vi "关键参数查询.vi"() -> ()   [LabVIEW 2016, in "斯坦道总磷.lvlib"]
panel:
  in  "参数下拉列表":u16(ring)
  out "关键参数":T1
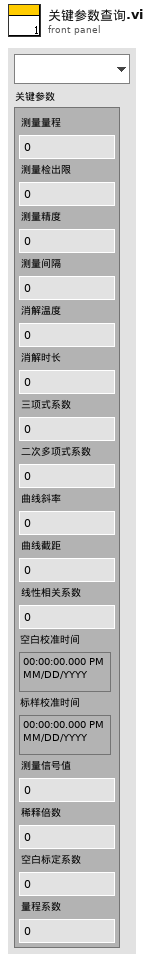
[diagram p1: front panel]
types:
  T1 = typedef "斯坦道总磷.lvlib/关键参数.ctl" = cluster{"测量量程":sgl, "测量检出限":sgl, "测量精度":sgl, "测量间隔":sgl, "消解温度":sgl, "消解时长":sgl, "三项式系数":sgl, "二次多项式系数":sgl, "曲线斜率":sgl, "曲线截距":sgl, "线性相关系数":sgl, "空白校准时间":timestamp, "标样校准时间":timestamp, "测量信号值":sgl, "稀释倍数":sgl, "空白标定系数":sgl, "量程系数":sgl}
  T2 = typedef "LVStringsAndValuesArrayTypeDef_U16.ctl" = cluster{"String":string, "Value":u16}[]
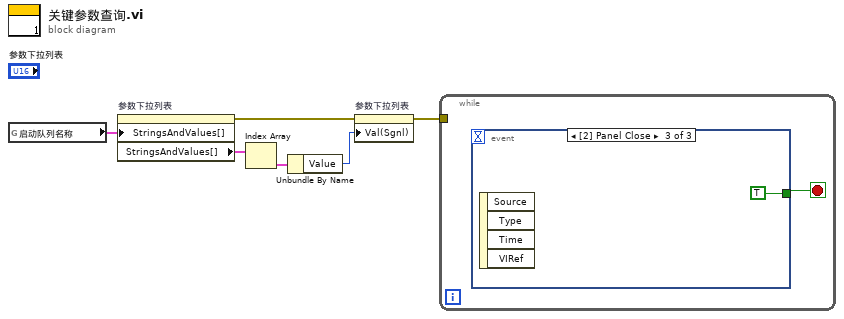
[diagram p0: block diagram]
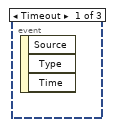
[diagram p2: hidden frame]
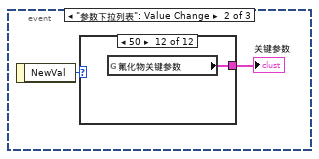
[diagram p3: hidden frame]
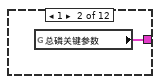
[diagram p5: hidden frame]
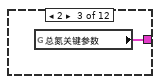
[diagram p6: hidden frame]
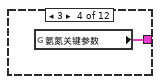
[diagram p7: hidden frame]
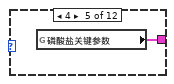
[diagram p8: hidden frame]
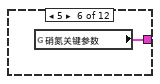
[diagram p9: hidden frame]
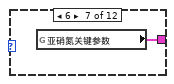
[diagram p10: hidden frame]
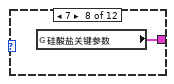
[diagram p11: hidden frame]
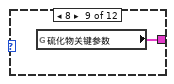
[diagram p12: hidden frame]
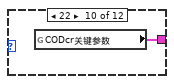
[diagram p13: hidden frame]
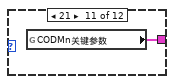
[diagram p14: hidden frame]
diagram:
  n1 = global read "model config var.vi" "启动队列名称"() -> (w2:cluster{"String":string, "Value":u16}[])
  n2 = property on="参数下拉列表" class="Ring (strict)"("StringsAndValues[]"=w2) -> (error out=w5:errorcluster, "StringsAndValues[]"=w3:T2)  [unwired: 2 in, 1 out]
  n3 = Index Array(array=w3) -> (element=w4:cluster{"String":string, "Value":u16})  [unwired: 1 in]
  n4 = Unbundle By Name(w4) -> ("Value"=w6:u16)
  n5 = property on="参数下拉列表" class="Ring (strict)"(error in=w5, "Val(Sgnl)"=w6) -> (error out=w1:errorcluster)  [unwired: 1 in, 1 out]
  n6 = while {
    tunnel: w1 -> [_]
    stop <- w7 stop-if-true
    n7 = event shown="[2] Panel Close" {
      selector: _ -> [_ _ _]
      dyn-events: _ -> [_ _ _]
      timeout: _ -> [_ _ _]
      tunnel: [_ _ TRUE] -> w7
      event Timeout {
        n8 = event-data() -> ()  [unwired: 1 in, 3 out]
      }
      event "参数下拉列表": Value Change {
        n9 = event-data() -> ("NewVal"=w9:u16)  [unwired: 1 in]
        n10 = case shown="50" w9 {
          tunnel: [_ w10 w11 w12 w13 w14 w15 w16 w17 w18 w19 w20] -> w8
          frame 0, Default {
          }
          frame 1 {
            n11 = global read "VAR总磷总氮全局变量.vi" "总磷关键参数"() -> (w10:T1)
          }
          frame 2 {
            n12 = global read "VAR总磷总氮全局变量.vi" "总氮关键参数"() -> (w11:T1)
          }
          frame 3 {
            n13 = global read "VAR总磷总氮全局变量.vi" "氨氮关键参数"() -> (w12:T1)
          }
          frame 4 {
            n14 = global read "VAR总磷总氮全局变量.vi" "磷酸盐关键参数"() -> (w13:T1)
          }
          frame 5 {
            n15 = global read "VAR总磷总氮全局变量.vi" "硝氮关键参数"() -> (w14:T1)
          }
          frame 6 {
            n16 = global read "VAR总磷总氮全局变量.vi" "亚硝氮关键参数"() -> (w15:T1)
          }
          frame 7 {
            n17 = global read "VAR总磷总氮全局变量.vi" "硅酸盐关键参数"() -> (w16:T1)
          }
          frame 8 {
            n18 = global read "VAR总磷总氮全局变量.vi" "硫化物关键参数"() -> (w17:T1)
          }
          frame 22 {
            n19 = global read "VAR总磷总氮全局变量.vi" "CODcr关键参数"() -> (w18:T1)
          }
          frame 21 {
            n20 = global read "VAR总磷总氮全局变量.vi" "CODMn关键参数"() -> (w19:T1)
          }
          frame 50 {
            n21 = global read "VAR总磷总氮全局变量.vi" "氟化物关键参数"() -> (w20:T1)
          }
        }
        "关键参数" <- w8
      }
      event Panel Close {
        n22 = event-data() -> ()  [unwired: 1 in, 4 out]
      }
    }
  }
